vi "mod_BB-PSK generation (one-shot).vi"(0 "Bit stream":T4(tab), 5 "PN Sequence Order":i32=9, 7 "Modulation specific parameters":T2={"filter parameters"={"Alpha"=0.5, "Filter Length"=8, "TX Filter"=enum."Root Raised Cos"}, "Symbol Rate, Hz"=100000.0, "PSK system parameters"={"samples per symbol (16)"=16, "symbol map"=[], "differential PSK"=enum."disable", "PSK type"=0}} {"PSK system parameters"."PSK type" items=["normal", "shifted", "offset"]; "PSK system parameters"."symbol map" format="%.3f"; "Symbol Rate, Hz" format="%.2p"; "filter parameters"."Alpha" format="%.2f"}, 9 "One-shot generation parameters":T3={"Enable channel coding? (T)"=FALSE, "Synchronization specific"={"Sync Number"=59786, "Sync bits"=16, "Sync Start Location, Symbols"=1}, "Channel coding specific"={"Channel coding type"=enum."Reed-Solomon encoding", "BCH parameters"={"n,k,t"="7,4,1"}, "Reed-Solomon parameters"={"code word length (n), symbols"=7, "data word length (k), symbols"=3}, "Golay parameters"={"Golay code type (n,k,t)"=enum."Golay (23,12,3)"}, "Convolutional parameters"={"rate (k/n)"=enum."1/2", "constraint length (K)"=3, "initial state"=0}}, "Message specific"={"Burst Length, Symbols"=500, "Burst Period, Symbols"=1000}} {"Channel coding specific"."Convolutional parameters"."initial state" format="%.0x"; "Synchronization specific"."Sync Number" format="%.0x"}, 11 "error in (no error)":errorcluster, 12 "user base bit pattern":i8[](array[numeric]), 13 "Path":path) -> (4 "output complex waveform":T5 {"Y" format="%.3f"; "dt" format="%^.2e"; "t0" format="%.4f"}, 15 "error out":errorcluster)   [LabVIEW 2020, in "niDMT.lvlib"]
uses:
  <vilib>/addons/Modulation/niDMT.lvlib
  <vilib>/addons/Modulation/Analog/controls/Complex Data Waveform.ctl
  <vilib>/addons/Modulation/Digital/Support/Controls/PSK System Parameters.ctl
  <vilib>/addons/Modulation/Digital/General/MT Generate Bits (Galois, PN Order).vi
  <vilib>/addons/Modulation/Digital/Channel Coding/MT Convolutional Encoder (Rate).vi
  <vilib>/addons/Modulation/Analog/support/mod_Set Error Source.vi
  <vilib>/addons/Modulation/Digital/Support/Common/Validators/mod_Generate Bits Validate.vi
  <vilib>/addons/Modulation/Digital/Support/Common/Validators/mod_Validate Bit Stream.vi
  <vilib>/addons/Modulation/Digital/Channel Coding/Convolutional codes/mod_Convolutional encoder.vi
  <vilib>/addons/Modulation/Digital/Channel Coding/Convolutional codes/subVIs/mod_Generate encoder tap connections.vi
  <vilib>/addons/Modulation/Digital/Channel Coding/Convolutional codes/subVIs/mod_Perform convolutional encoding.vi
  <vilib>/addons/Modulation/Digital/Channel Coding/Block codes/subVIs/mod_Buffer block code info (I8).vi
  <vilib>/addons/Modulation/Digital/Channel Coding/Convolutional codes/subVIs/mod_Generate valid reset (convolutional, I8).vi
  <vilib>/Utility/file.llb/Read From Spreadsheet File (DBL).vi
  <vilib>/addons/Modulation/Digital/Support/Common/Validators/mod_Generate Filter Coefficients Validate.vi
  <vilib>/addons/Modulation/Digital/General/subVIs/mod_Generate Filter Coefficients.vi
  <vilib>/addons/Modulation/Digital/General/subVIs/mod_Generate Bits PN Sequence.vi
  <vilib>/addons/Modulation/Digital/General/MT Generate Bits (User Defined).vi
  <vilib>/addons/Modulation/Digital/Channel Coding/MT BCH Encoder (Systematic).vi
  <vilib>/addons/Modulation/Digital/Channel Coding/MT RS Symbol Encoder (normal).vi
  <vilib>/addons/Modulation/Digital/Channel Coding/Convolutional codes/subVIs/mod_Select known generator matrix.vi
  <vilib>/addons/Modulation/Digital/Support/Common/Validators/mod_Validate Convolutional Encoder prms.vi
  <resource>/objmgr/NIMTAttribs.rc
  <vilib>/addons/Modulation/niAMT.lvlib
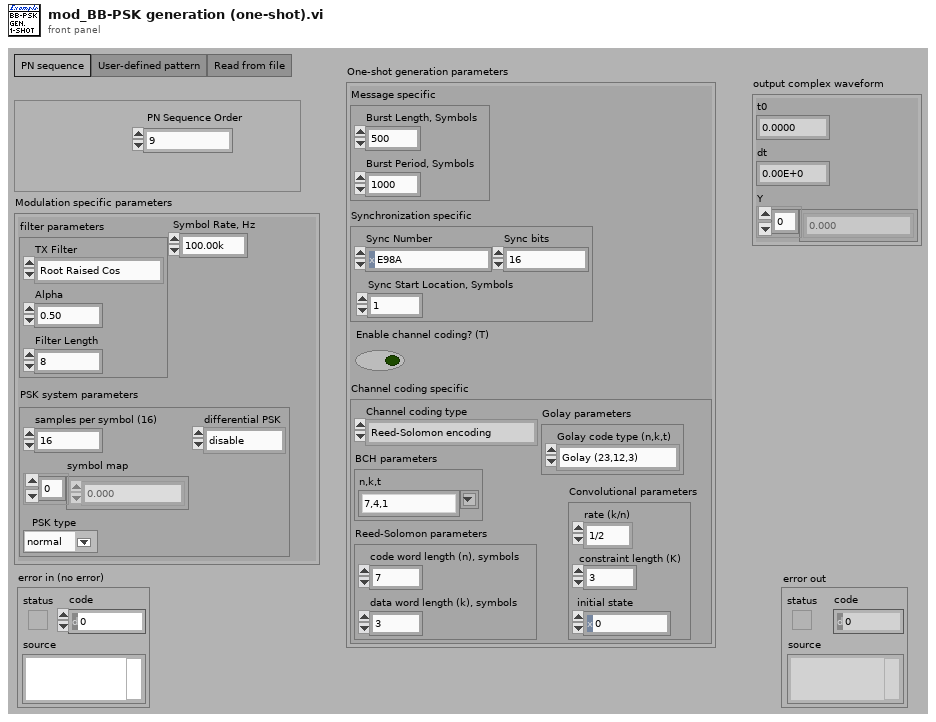
[diagram p1: front panel]
types:
  T1 = typedef "niDMT.lvlib/PSK System Parameters.ctl" = cluster{"samples per symbol (16)":i32, "symbol map":cdb[], "differential PSK":enum16{"disable", "enable"}, "PSK type":u16}
  T2 = cluster{"filter parameters":cluster{"Alpha":dbl, "Filter Length":i32, "TX Filter":enum16{"none", "Raised Cosine", "Root Raised Cos", "Gaussian"}}, "Symbol Rate, Hz":dbl, "PSK system parameters":T1}
  T3 = cluster{"Enable channel coding? (T)":bool, "Synchronization specific":cluster{"Sync Number":u32, "Sync bits":i32, "Sync Start Location, Symbols":i32}, "Channel coding specific":cluster{"Channel coding type":enum16{"BCH encoding", "Reed-Solomon encoding", "Convolutional encoding", "Golay encoding"}, "BCH parameters":cluster{"n,k,t":string}, "Reed-Solomon parameters":cluster{"code word length (n), symbols":i32, "data word length (k), symbols":i32}, "Golay parameters":cluster{"Golay code type (n,k,t)":enum16{"Golay (23,12,3)", "Golay (24,12,3)"}}, "Convolutional parameters":cluster{"rate (k/n)":enum16{"1/2", "1/3", "1/4", "2/3", "3/4"}, "constraint length (K)":i32, "initial state":u32}}, "Message specific":cluster{"Burst Length, Symbols":i32, "Burst Period, Symbols":i32}}
  T4 = enum32{"PN sequence", "User-defined pattern", "Read from file"}
  T5 = typedef "niAMT.lvlib/Complex Data Waveform.ctl" = cluster{"t0":dbl, "dt":dbl, "Y":cdb[]}
  T6 = enum16{"none", "Raised Cosine", "Root Raised Cos", "Gaussian"}
  T7 = cluster{"Sync Number":u32, "Sync bits":i32, "Sync Start Location, Symbols":i32}
  T8 = enum16{"BCH encoding", "Reed-Solomon encoding", "Convolutional encoding", "Golay encoding"}
  T9 = typedef "niDMT.lvlib/MT Generic Refnum.ctl" = refnum<k20>
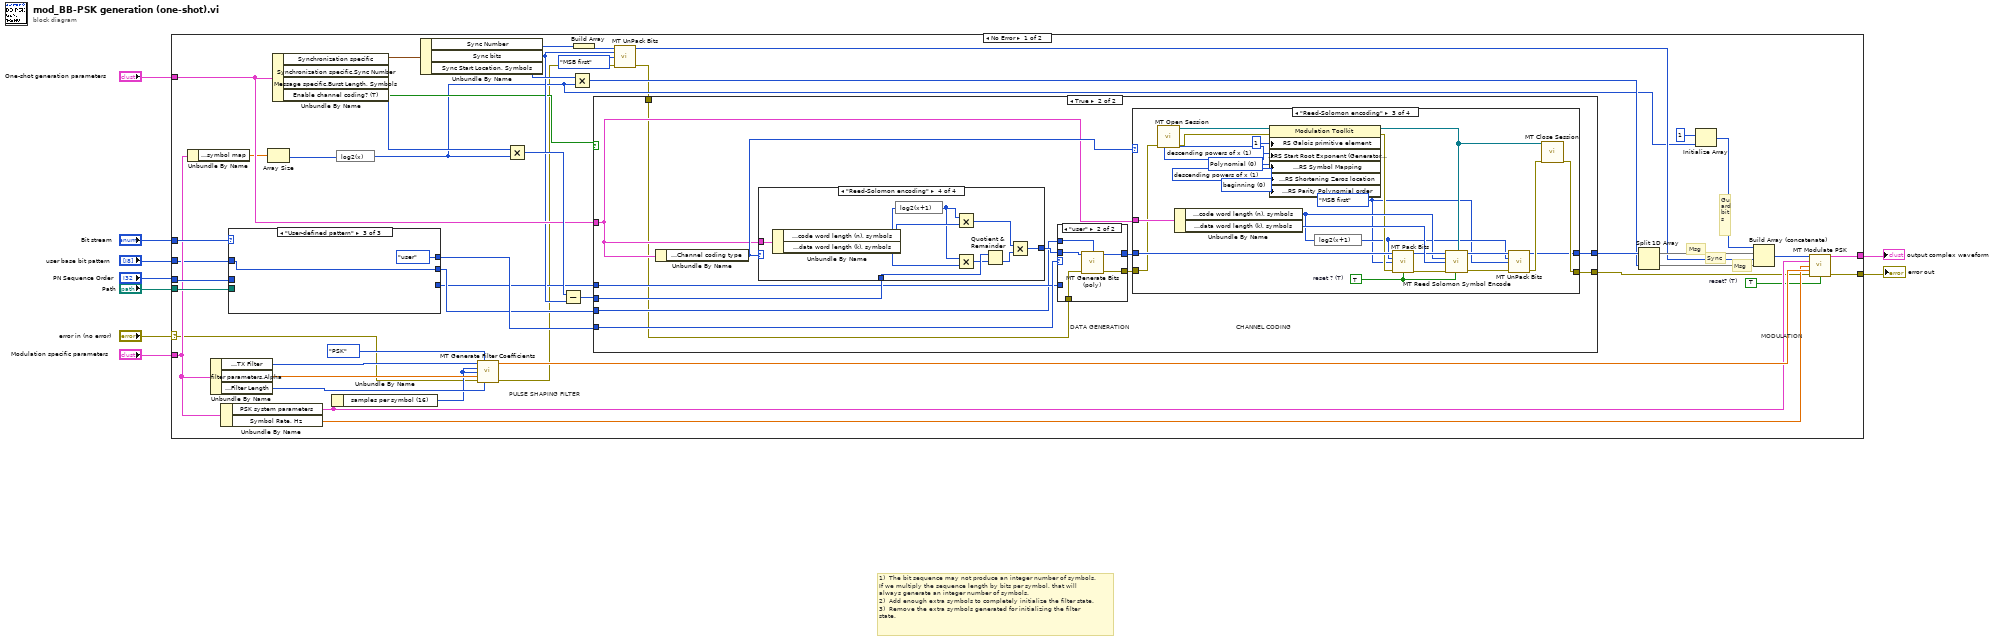
[diagram p0: block diagram]
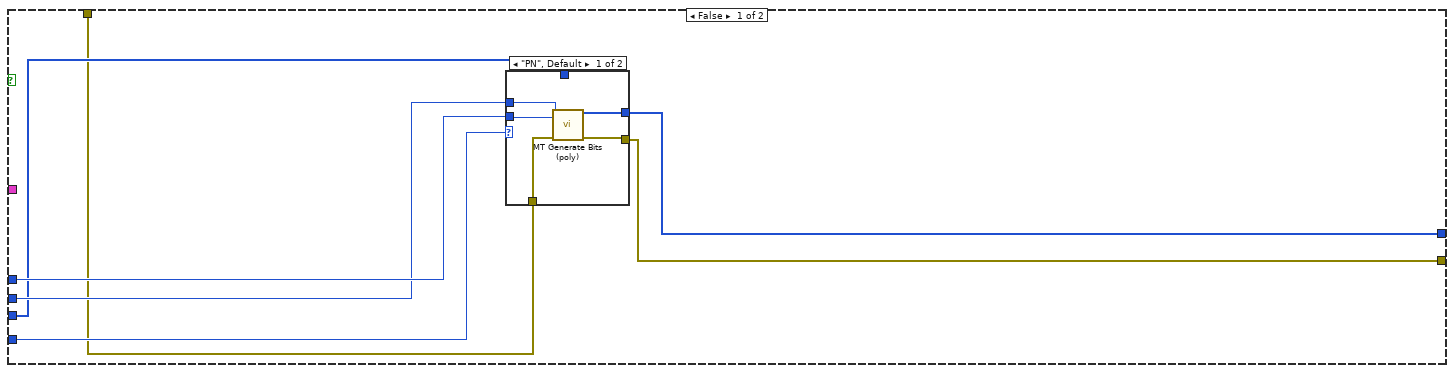
[diagram p2: hidden frame]
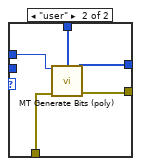
[diagram p3: hidden frame]
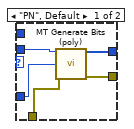
[diagram p4: hidden frame]
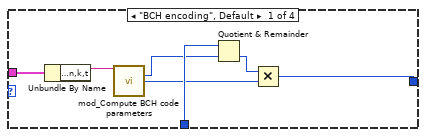
[diagram p5: hidden frame]
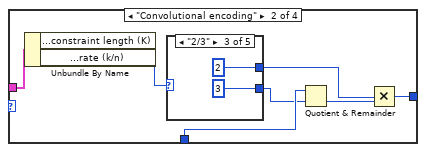
[diagram p6: hidden frame]
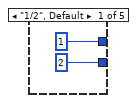
[diagram p7: hidden frame]
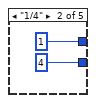
[diagram p8: hidden frame]
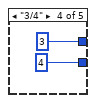
[diagram p9: hidden frame]
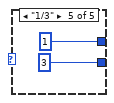
[diagram p10: hidden frame]
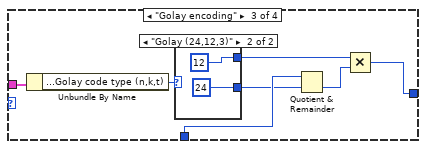
[diagram p11: hidden frame]
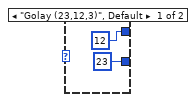
[diagram p12: hidden frame]
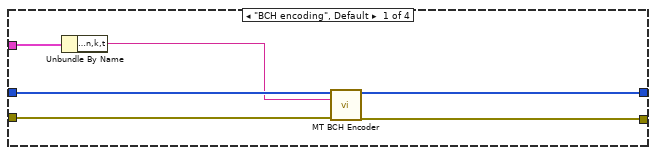
[diagram p13: hidden frame]
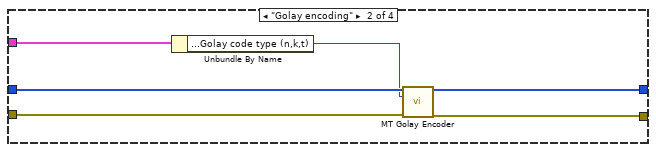
[diagram p14: hidden frame]
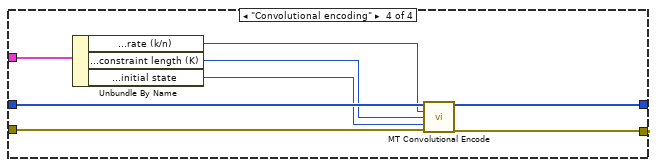
[diagram p15: hidden frame]
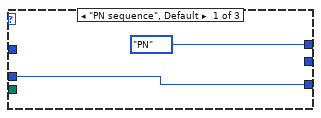
[diagram p16: hidden frame]
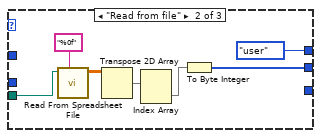
[diagram p17: hidden frame]
diagram:
  # "1)  The bit sequence may not produce an integer number of symbols.  If we multiply the sequence length by bits per symbol, that will always generate an integer number of symbols. \n2)  Add enough extra symbols to completely initialize the filter state.\n3)  Remove the extra symbols generated for initializing the filter state."
  n1 = case shown="No Error" "error in (no error)" {
    selector: "error in (no error)" -> [w13 w193]
    tunnel: [w54 w193] -> w9
    tunnel: "PN Sequence Order" -> [w46 _]
    tunnel: "Bit stream" -> [w48 _]
    tunnel: "Modulation specific parameters" -> [w29 _]
    tunnel: "Path" -> [w47 _]
    tunnel: "One-shot generation parameters" -> [w42 _]
    tunnel: [w27 _] -> w3
    tunnel: "user base bit pattern" -> [w21 _]
    frame No Error {
      w14 = TRUE  # reset? (T)
      # "PULSE SHAPING FILTER"
      # "MODULATION"
      # "Msg"
      # "Sync"
      # "Msg"
      # "Guard bits"
      n2 = Unbundle By Name(w29) -> ("PSK system parameters.symbol map"=w26:cdb[])
      n3 = Unbundle By Name(w29) -> ("filter parameters.TX Filter"=w51:T6, "filter parameters.Alpha"=w53:dbl, "filter parameters.Filter Length"=w52:i32)
      n4 = Unbundle By Name(w29) -> ("PSK system parameters"=w23:T1, "Symbol Rate, Hz"=w28:dbl)
      n5 = case shown="\"User-defined pattern\"" w48 {
        tunnel: [_ w185 w191] -> w40
        tunnel: [enum16{"PN", "user"}."PN" ("mode (PN)") enum16{"PN", "user"}."user" ("mode (PN)") enum16{"PN", "user"}."user" ("mode (PN)")] -> w41
        tunnel: w46 -> [w182 _ _]
        tunnel: w47 -> [_ w187 _]
        tunnel: w21 -> [_ _ w191]
        tunnel: [w182 _ _] -> w20
        frame "PN sequence", Default {
        }
        frame "Read from file" {
          n6 = call-poly <vilib>:"Read From Spreadsheet File.vi"("format (%.3f)"="%0f", "file path (dialog if empty)"=w187) -> ("all rows"=w188:dbl[][])  [unwired: 2 in, 7 out]
          n7 = Transpose 2D Array(2D array=w188) -> (transposed array=w189:dbl[][])
          n8 = Index Array(array=w189) -> (element=w190:dbl[])  [unwired: 2 in]
          n9 = To Byte Integer(number=w190) -> (8bit integer=w185:i8[])
        }
        frame "User-defined pattern" {
        }
      }
      n10 = Array Size(array=w26) -> (size(s)=w25:i32)
      n11 = Unbundle By Name(w42) -> ("Synchronization specific"=w39:T7, "Message specific.Burst Length, Symbols"=w45:i32, "Enable channel coding? (T)"=w35:bool)  [unwired: 1 out]
      n12 = Unbundle By Name(w23) -> ("samples per symbol (16)"=w22:i32)
      n13 = expression code="log2(x)"(w25) -> (w18:i32)
      n14 = Unbundle By Name(w39) -> ("Sync Number"=w16:u32, "Sync bits"=w36:i32, "Sync Start Location, Symbols"=w37:i32)
      n15 = call <vilib>:"MT Generate Filter Coefficients.vi"("pulse shaping filter (none)"=w51, "modulation type"=enum16{"FSK", "PSK", "QAM", "MSK", "PAM", "ASK"}."PSK", "pulse shaping samples per symbol (16)"=w22, "matched samples per symbol (16)"=w22, "filter parameter"=w53, "error in (no error)"=w13, "filter length (symbols)"=w52) -> ("pulse shaping filter coefficients"=w50:dbl[], "error out"=w11:errorcluster)  [unwired: 7 out]
      n16 = Multiply(x=w45, y=w18) -> (x*y=w44:i32)
      n17 = Subtract(x=w44, y=w36) -> (x-y=w43:i32)
      n18 = Multiply(x=w37, y=w18) -> (x*y=w34:i32)
      n19 = Build Array(w16) -> (w15:u32[])
      n20 = call <vilib>:"MT UnPack Bits.vi"("input integers"=w15, "bits per integer"=w36, "packed bit order"=enum16{"MSB first", "LSB first"}."MSB first" ("bit order"), "error in (no error)"=w11) -> ("output bit stream"=w32:i8[], "error out"=w10:errorcluster)  [unwired: 1 in, 9 out]
      n21 = case shown="True" w35 {
        tunnel: w43 -> [w59 w82]
        tunnel: w42 -> [_ w80]
        tunnel: w41 -> [w61 w78]
        tunnel: w40 -> [w56 w73]
        tunnel: [w57 w81] -> w38
        tunnel: [w58 w79] -> w12
        tunnel: w20 -> [w60 w76]
        tunnel: w10 -> [w55 w72]
        frame False {
          n22 = case shown="\"PN\", Default" w61 {
            tunnel: w60 -> [w66 _]
            tunnel: w59 -> [w65 w70]
            tunnel: w55 -> [w64 w69]
            tunnel: [w63 w67] -> w58
            tunnel: [w62 w68] -> w57
            tunnel: w56 -> [_ w71]
            frame "PN", Default {
              n23 = call-poly <vilib>:"MT Generate Bits (poly).vi"("total bits (128)"=w65, "PN sequence order (9)"=w66, "error in (no error)"=w64) -> ("output bit stream"=w62:i8[], "error out"=w63:errorcluster)  [unwired: 2 in, 9 out]
            }
            frame "user" {
              n24 = call-poly <vilib>:"MT Generate Bits (poly).vi"("total bits (128)"=w70, "user base bit pattern"=w71, "error in (no error)"=w69) -> ("output bit stream"=w68:i8[], "error out"=w67:errorcluster)  [unwired: 1 in, 10 out]
            }
          }
        }
        frame True {
          # "CHANNEL CODING"
          # "DATA GENERATION"
          n25 = Unbundle By Name(w80) -> ("Channel coding specific.Channel coding type"=w83:T8)
          n26 = case shown="\"Reed-Solomon encoding\"" w83 {
            tunnel: w80 -> [w100 w107 w124 w137]
            tunnel: w82 -> [w98 w105 w121 w133]
            tunnel: [w94 w102 w118 w130] -> w77
            frame "BCH encoding", Default {
              n27 = Unbundle By Name(w100) -> ("Channel coding specific.BCH parameters.n,k,t"=w99:string)
              n28 = call <vilib>:"mod_Compute BCH code parameters.vi"("n,k,t"=w99) -> ("n"=w97:i32, "k"=w95:i32)  [unwired: 2 in, 11 out]
              n29 = Quotient & Remainder(x=w98, y=w97) -> (floor(x/y)=w96:i32)  [unwired: 1 out]
              n30 = Multiply(x=w96, y=w95) -> (x*y=w94:i32)
            }
            frame "Convolutional encoding" {
              n31 = Unbundle By Name(w107) -> ("Channel coding specific.Convolutional parameters.rate (k/n)"=w106:enum16{"1/2", "1/3", "1/4", "2/3", "3/4"})  [unwired: 1 out]
              n32 = case shown="\"2/3\"" w106 {
                tunnel: [2 4 3 4 3] -> w103
                tunnel: [1 1 2 3 1] -> w101
                frame "1/2", Default {
                }
                frame "1/4" {
                }
                frame "2/3" {
                }
                frame "3/4" {
                }
                frame "1/3" {
                }
              }
              n33 = Quotient & Remainder(x=w105, y=w103) -> (floor(x/y)=w104:i32)  [unwired: 1 out]
              n34 = Multiply(x=w101, y=w104) -> (x*y=w102:i32)
            }
            frame "Golay encoding" {
              n35 = Unbundle By Name(w124) -> ("Channel coding specific.Golay parameters.Golay code type (n,k,t)"=w123:enum16{"Golay (23,12,3)", "Golay (24,12,3)"})
              n36 = case shown="\"Golay (24,12,3)\"" w123 {
                tunnel: [23 24] -> w120
                tunnel: [12 12] -> w119
                frame "Golay (23,12,3)", Default {
                }
                frame "Golay (24,12,3)" {
                }
              }
              n37 = Quotient & Remainder(x=w121, y=w120) -> (floor(x/y)=w122:i32)  [unwired: 1 out]
              n38 = Multiply(x=w119, y=w122) -> (x*y=w118:i32)
            }
            frame "Reed-Solomon encoding" {
              n39 = Unbundle By Name(w137) -> ("Channel coding specific.Reed-Solomon parameters.code word length (n), symbols"=w136:i32, "Channel coding specific.Reed-Solomon parameters.data word length (k), symbols"=w135:i32)
              n40 = expression code="log2(x+1)"(w136) -> (w129:i32)
              n41 = Multiply(x=w129, y=w135) -> (x*y=w131:i32)
              n42 = Multiply(x=w129, y=w136) -> (x*y=w132:i32)
              n43 = Quotient & Remainder(x=w133, y=w132) -> (floor(x/y)=w134:i32)  [unwired: 1 out]
              n44 = Multiply(x=w131, y=w134) -> (x*y=w130:i32)
            }
          }
          n45 = case shown="\"user\"" w78 {
            tunnel: w77 -> [w88 w93]
            tunnel: w76 -> [w87 _]
            tunnel: w72 -> [w86 w91]
            tunnel: [w85 w90] -> w75
            tunnel: [w84 w89] -> w74
            tunnel: w73 -> [_ w92]
            frame "PN", Default {
              n46 = call-poly <vilib>:"MT Generate Bits (poly).vi"("total bits (128)"=w88, "PN sequence order (9)"=w87, "error in (no error)"=w86) -> ("output bit stream"=w84:i8[], "error out"=w85:errorcluster)  [unwired: 2 in, 9 out]
            }
            frame "user" {
              n47 = call-poly <vilib>:"MT Generate Bits (poly).vi"("total bits (128)"=w93, "user base bit pattern"=w92, "error in (no error)"=w91) -> ("output bit stream"=w89:i8[], "error out"=w90:errorcluster)  [unwired: 1 in, 10 out]
            }
          }
          n48 = case shown="\"Reed-Solomon encoding\"" w83 {
            tunnel: w74 -> [w141 w149 w171 w181]
            tunnel: w75 -> [w143 w148 w161 w180]
            tunnel: [w142 w147 w159 w178] -> w79
            tunnel: [w140 w144 w153 w179] -> w81
            tunnel: w80 -> [w139 w146 w173 w177]
            frame "BCH encoding", Default {
              n49 = Unbundle By Name(w139) -> ("Channel coding specific.BCH parameters.n,k,t"=w138:string)
              n50 = call-poly <vilib>:"MT BCH Encoder.vi"("input bit stream"=w141, "n,k,t"=w138, "error in (no error)"=w143) -> ("output bit stream"=w140:i8[], "error out"=w142:errorcluster)  [unwired: 1 in, 10 out]
            }
            frame "Golay encoding" {
              n51 = Unbundle By Name(w146) -> ("Channel coding specific.Golay parameters.Golay code type (n,k,t)"=w145:enum16{"Golay (23,12,3)", "Golay (24,12,3)"})
              n52 = call <vilib>:"MT Golay Encoder.vi"("input bit stream"=w149, "Golay code type (n,k,t)"=w145, "error in (no error)"=w148) -> ("output bit stream"=w144:i8[], "error out"=w147:errorcluster)  [unwired: 1 in, 10 out]
            }
            frame "Reed-Solomon encoding" {
              w151 = enum16{"MSB first", "LSB first"}."MSB first" ("packed bit order")
              w150 = 0 items=["Polynomial", "Exponent"] ("Channel Coding:Reed Solomon:RS Symbol Mapping")
              w162 = 0 items=["beginning", "end"] ("Channel Coding:Reed Solomon:RS Parity Position")
              w163 = 1 items=["ascending powers of x", "descending powers of x"] ("Channel Coding:Reed Solomon:RS Parity Polynomial order")
              w164 = 1 items=["ascending powers of x", "descending powers of x"] ("Channel Coding:Reed Solomon: RS Message Polynomial order")
              w157 = TRUE  # reset ? (T)
              n53 = call <vilib>:"MT Open Session.vi"("error in (no error)"=w161) -> ("modulation session"=w167:T9, "error out"=w166:errorcluster)  [unwired: 13 out]
              n54 = Unbundle By Name(w173) -> ("Channel coding specific.Reed-Solomon parameters.code word length (n), symbols"=w168:i32, "Channel coding specific.Reed-Solomon parameters.data word length (k), symbols"=w172:i32)
              n55 = property class="Modulation Toolkit"(reference=w167, error in=w166, "RS Galois primitive element"=1 ("Channel Coding:Reed Solomon: RS Start Root Exponent (Generator Polynomial)"), "Channel Coding:Reed Solomon:RS Start Root Exponent (Generator Polynomial)"=w164, "Channel Coding:Reed Solomon:RS Symbol Mapping"=w150, "Channel Coding:Reed Solomon:RS Shortening Zeros location"=w163, "Channel Coding:Reed Solomon:RS Parity Polynomial order"=w162) -> (reference out=w158:T9, error out=w160:errorcluster)
              n56 = expression code="log2(x+1)"(w168) -> (w152:i32)
              n57 = call <vilib>:"MT Pack Bits.vi"("input bit stream"=w171, "bits per integer"=w152, "packed bit order"=w151, "error in (no error)"=w160, "reset ? (T)"=w157) -> ("output integers"=w170:i32[], "error out"=w169:errorcluster)  [unwired: 1 in, 8 out]
              n58 = call-poly <vilib>:"MT Reed Solomon Symbol Encode.vi"("input symbols"=w170, "modulation session"=w158, "code word length (n), symbols"=w168, "data word length (k), symbols"=w172, "error in (no error)"=w169, "reset? (T)"=w157) -> ("output symbols"=w156:i32[], "error out"=w155:errorcluster)  [unwired: 8 out]
              n59 = call <vilib>:"MT UnPack Bits.vi"("input integers"=w156, "bits per integer"=w152, "packed bit order"=w151, "error in (no error)"=w155) -> ("output bit stream"=w153:i8[], "error out"=w154:errorcluster)  [unwired: 1 in, 9 out]
              n60 = call <vilib>:"MT Close Session.vi"("modulation session"=w158, "error in (no error)"=w154) -> ("error out"=w159:errorcluster)  [unwired: 13 out]
            }
            frame "Convolutional encoding" {
              n61 = Unbundle By Name(w177) -> ("Channel coding specific.Convolutional parameters.rate (k/n)"=w176:enum16{"1/2", "1/3", "1/4", "2/3", "3/4"}, "Channel coding specific.Convolutional parameters.constraint length (K)"=w175:i32, "Channel coding specific.Convolutional parameters.initial state"=w174:u32)
              n62 = call-poly <vilib>:"MT Convolutional Encode.vi"("input bit stream"=w181, "rate (k/n)"=w176, "constraint length (K)"=w175, "initial state"=w174, "error in (no error)"=w180) -> ("output bit stream"=w179:i8[], "error out"=w178:errorcluster)  [unwired: 1 in, 8 out]
            }
          }
        }
      }
      n63 = Split 1D Array(array=w38, index=w34) -> (first subarray=w33:i8[], second subarray=w31:i8[])
      n64 = Initialize Array(i8 1 ("element"), w18) -> (w17:i8[])
      n65 = Build Array (concatenate)(w17, w33, w32, w31) -> (w30:i8[])
      n66 = call <vilib>:"MT Modulate PSK.vi"("input bit stream"=w30, "PSK system parameters"=w23, "symbol rate (Hz)"=w28, "pulse shaping filter coefficients"=w50, "error in (no error)"=w12, "reset? (T)"=w14) -> ("output complex waveform"=w27:T5, "error out"=w54:errorcluster)  [unwired: 1 in, 7 out]
    }
    frame Error {
    }
  }
  "error out" <- w9
  "output complex waveform" <- w3
